vi "roi_to_FPGA_points.vi"(8 "error in":errorcluster, 9 "z in":u16[](array[numeric]), 10 "amplitude in":u16[](array[numeric]), 11 "TrajectoryMG100122AODFrameScan in":refnum<class "TrajectoryMH100122AODRAPS.lvclass">) -> (0 "error out":errorcluster, 3 "TrajectoryMG100122AODFrameScan out":refnum<class "TrajectoryMH100122AODRAPS.lvclass">)   [LabVIEW 2010, in "TrajectoryMH100122AODRAPS.lvclass"]
uses:
  TrajectoryMH100122AODRAPS.lvclass
  common/xcontrols/XImage/XImage/XImage.xctl
  TrajectoryMH100122AODRAPS.lvclass/TrajectoryMH100122AODRAPS.ctl
  class_data.vi
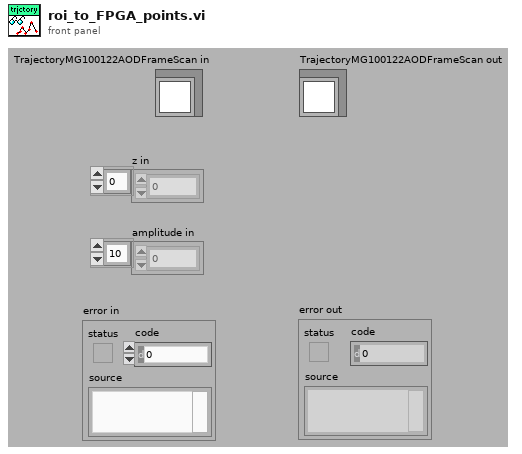
[diagram p1: front panel]
types:
  T1 = cluster{"Global Rectangle":i32[], "Contours":cluster{"Contour Type":u32, "ROI Type":u32, "Points":i32[]}[]}[]
  T2 = cluster{"Contour Type":u32, "ROI Type":u32, "Points":i32[]}[]
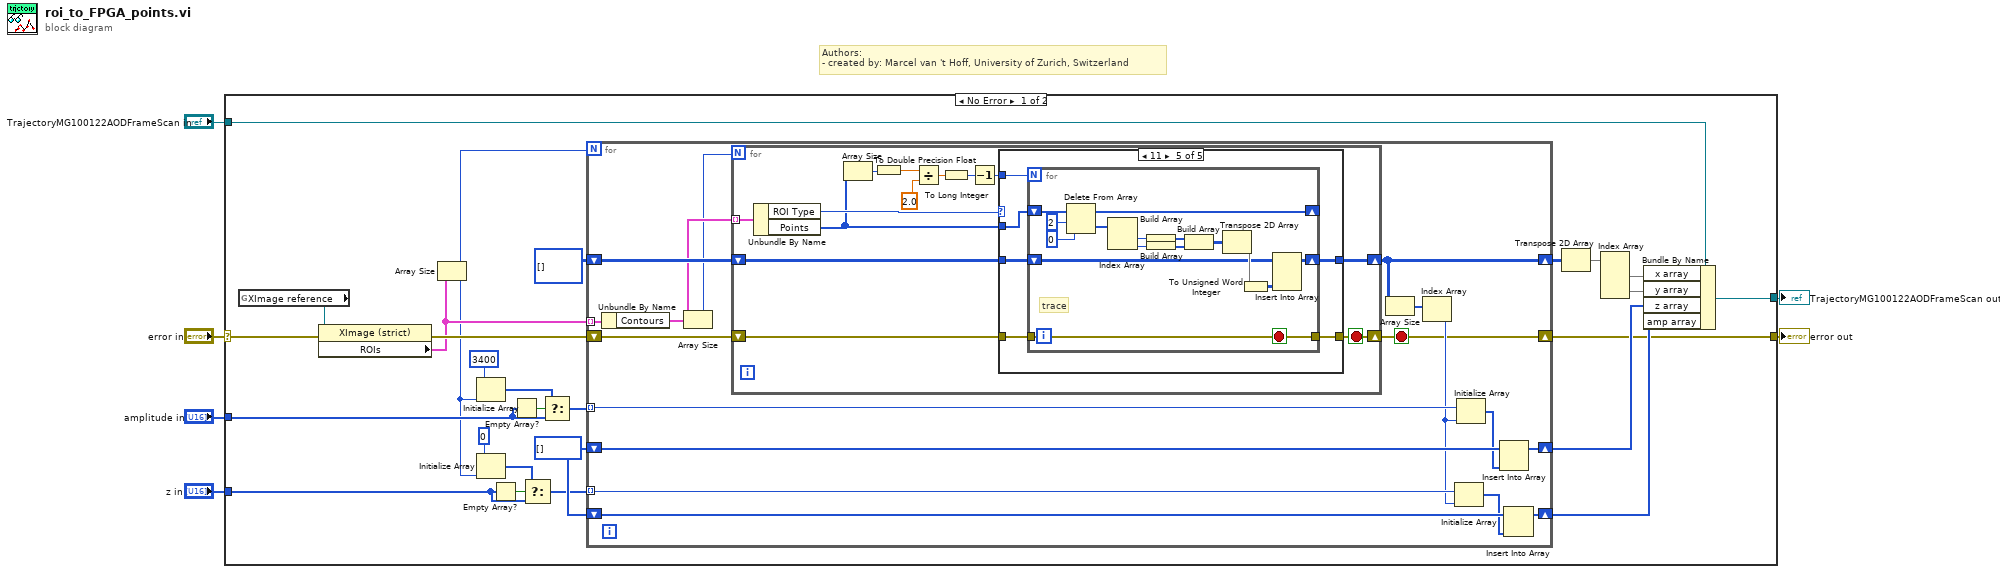
[diagram p0: block diagram]
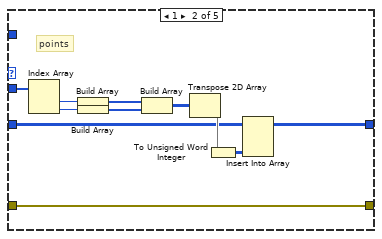
[diagram p3: hidden frame]
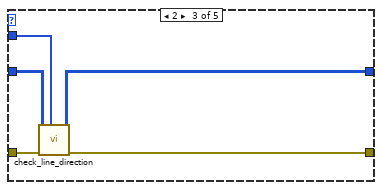
[diagram p4: hidden frame]
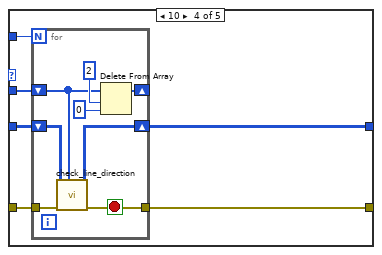
[diagram p5: hidden frame]
diagram:
  # "Authors: \n- created by: Marcel van 't Hoff, University of Zurich, Switzerland"
  n1 = case shown="No Error" "error in" {
    selector: "error in" -> [w21 w117]
    tunnel: [w24 w117] -> w6
    tunnel: "amplitude in" -> [w16 _]
    tunnel: "z in" -> [w10 _]
    tunnel: "TrajectoryMG100122AODFrameScan in" -> [w18 w116]
    tunnel: [w23 w116] -> w3
    frame No Error {
      w26 = u16[] []
      n2 = global read "class_data.vi" "XImage reference"() -> (w22:refnum<vi>)
      n3 = property class="XImage (strict)"(reference=w22, error in=w21) -> (error out=w20:errorcluster, "ROIs"=w19:T1)  [unwired: 1 out]
      n4 = Array Size(array=w19) -> (size(s)=w9:i32)
      n5 = Initialize Array(u16 3400 ("element"), w9) -> (w13:u16[])
      n6 = Initialize Array(u16 0 ("element"), w9) -> (w8:u16[])
      n7 = Empty Array?(array=w10) -> (empty?=w11:bool)
      n8 = Empty Array?(array=w16) -> (empty?=w17:bool)
      n9 = Select(t=w8, s=w11, f=w10) -> (s? t:f=w7:u16[])
      n10 = Select(t=w13, s=w17, f=w16) -> (s? t:f=w15:u16[])
      n11 = for {
        N: w9 -> [_]
        tunnel: w19 -> [w49] mode=indexing
        shift-right: [w36] -> w31
        shift-left: u16[][] [] -> [w47]
        tunnel: w15 -> [w46] mode=indexing
        shift-right: [w43] -> w27
        shift-left: w26 -> [w45]
        tunnel: w7 -> [w41] mode=indexing
        shift-right: [w39] -> w25
        shift-left: w26 -> [w40]
        shift-right: [w33] -> w24
        shift-left: w20 -> [w48]
        stop <- w33 stop-if-true
        n12 = Unbundle By Name(w49) -> ("Contours"=w42:T2)
        n13 = Array Size(array=w42) -> (size(s)=w37:i32)
        n14 = for {
          N: w37 -> [_]
          tunnel: w42 -> [w62] mode=indexing
          shift-right: [w58] -> w36
          shift-left: w47 -> [w59]
          shift-right: [w60] -> w33
          shift-left: w48 -> [w61]
          stop <- w60 stop-if-true
          n15 = Unbundle By Name(w62) -> ("ROI Type"=w52:u32, "Points"=w50:i32[])
          n16 = Array Size(array=w50) -> (size(s)=w56:i32)
          n17 = To Double Precision Float(number=w56) -> (double precision float=w57:dbl)
          n18 = Divide(x=w57, y=2.0 ("length")) -> (x/y=w54:dbl)
          n19 = To Long Integer(number=w54) -> (32bit integer=w55:i32)
          n20 = Decrement(x=w55) -> (x-1=w51:i32)
          n21 = case shown="11" w52 {
            tunnel: w50 -> [_ w75 w76 w84 w98]
            tunnel: [w64 w74 w77 w82 w96] -> w60
            tunnel: w61 -> [w64 w74 w78 w83 w97]
            tunnel: w59 -> [w63 w67 w80 w86 w100]
            tunnel: [w63 w66 w79 w85 w99] -> w58
            tunnel: w51 -> [_ _ _ w81 w95]
            frame 0, Default {
            }
            frame 1 {
              # "points"
              n22 = Index Array(array=w75) -> (element #1=w73:i32, element #2=w72:i32)  [unwired: 2 in]
              n23 = Build Array(w73) -> (w71:i32[])
              n24 = Build Array(w72) -> (w70:i32[])
              n25 = Build Array(w71, w70) -> (w69:i32[][])
              n26 = Transpose 2D Array(2D array=w69) -> (transposed array=w68:i32[][])
              n27 = To Unsigned Word Integer(number=w68) -> (unsigned 16bit integer=w65:u16[][])
              n28 = Insert Into Array(array=w67, new element=w65) -> (w66:u16[][])  [unwired: 2 in]
            }
            frame 2 {
              n29 = call "check_line_direction.vi"("roi points in"=w76, "error in"=w78, "final array in"=w80) -> ("error out"=w77:errorcluster, "Array"=w79:u16[][])  [unwired: 7 in]
            }
            frame 10 {
              n30 = for {
                N: w81 -> [_]
                shift-right: [w90] -> w85
                shift-left: w86 -> [w91]
                tunnel: w83 -> [w89]
                tunnel: [w88] -> w82
                shift-right: [w92] -> _
                shift-left: w84 -> [w87]
                stop <- w88 stop-if-true
                n31 = call "check_line_direction.vi"("roi points in"=w87, "error in"=w89, "final array in"=w91) -> ("error out"=w88:errorcluster, "Array"=w90:u16[][])  [unwired: 7 in]
                n32 = Delete From Array(array=w87, length=2, index=0) -> (array with subset deleted=w92:i32[])  [unwired: 1 out]
              }
            }
            frame 11 {
              n33 = for {
                N: w95 -> [_]
                shift-right: [w108] -> w99
                shift-left: w100 -> [w109]
                shift-right: [w103] -> _
                shift-left: w98 -> [w107]
                tunnel: w97 -> [w102]
                tunnel: [w102] -> w96
                stop <- w102 stop-if-true
                # "trace"
                n34 = Delete From Array(array=w107, length=2, index=0) -> (deleted portion=w104:i32[], array with subset deleted=w103:i32[])
                n35 = Index Array(array=w104) -> (element #1=w115:i32, element #2=w114:i32)  [unwired: 2 in]
                n36 = Build Array(w115) -> (w113:i32[])
                n37 = Build Array(w114) -> (w112:i32[])
                n38 = Build Array(w113, w112) -> (w111:i32[][])
                n39 = Transpose 2D Array(2D array=w111) -> (transposed array=w110:i32[][])
                n40 = To Unsigned Word Integer(number=w110) -> (unsigned 16bit integer=w101:u16[][])
                n41 = Insert Into Array(array=w109, new element=w101) -> (w108:u16[][])  [unwired: 2 in]
              }
            }
          }
        }
        n42 = Array Size(array=w36) -> (size(s)=w35:i32[])
        n43 = Index Array(array=w35) -> (element=w34:i32)  [unwired: 1 in]
        n44 = Initialize Array(w41, w34) -> (w38:u16[])
        n45 = Initialize Array(w46, w34) -> (w44:u16[])
        n46 = Insert Into Array(array=w45, new element=w44) -> (w43:u16[])  [unwired: 1 in]
        n47 = Insert Into Array(array=w40, new element=w38) -> (w39:u16[])  [unwired: 1 in]
      }
      n48 = Transpose 2D Array(2D array=w31) -> (transposed array=w28:u16[][])
      n49 = Index Array(array=w28) -> (element #1=w30:u16[], element #2=w29:u16[])  [unwired: 4 in]
      n50 = Bundle By Name(cluster=w18, "x array"=w30, "y array"=w29, "z array"=w27, "amp array"=w25) -> (w23:refnum<class "TrajectoryMH100122AODRAPS.lvclass">)
    }
    frame Error {
    }
  }
  "error out" <- w6
  "TrajectoryMG100122AODFrameScan out" <- w3
